vi "DAQmx Data Acquisition.vi"(7 "measure call context in":refnum<class "Measure Call Context.lvclass">, 8 "error in":errorcluster, 11 "DAQmx Cfg":T1={"Run Mode"=0, "Sample Rate (Hz)"=51200.0, "Block Size"=5120, "Channel Table"=[], "Trigger Type"=0, "Trigger Channel"="", "Level"=0.0, "Pretrigger"=20, "Hysteresis"=0.0, "Slope"=enum."Rising"} {"Run Mode" items=["Run Once", "Continuously"]; "Block Size" min=0; "Sample Rate (Hz)" min=0.0; "Trigger Type" items=["None", "Analog Reference"]; "Channel Table"."input terminal configuration" items=["default"=-1, "RSE"=10083, "NRSE"=10078, "Differential"=10106, "Pseudodifferential"=12529]; "Channel Table"."Channel Type" items=["Voltage (V)"=0, "Charge (C)"=9, "-"=99, "SPL (Pa)"=3, "Force (lbf)"=6, "Force (N)"=1, "Acceleration (g) - IEPE"=2, "Acceleration (g) - Charge"=12, "Acceleration (g) - 4 wire DC Voltage"=22, "Velocity (in/s)"=7, "Velocity (mm/s)"=8, "Prox Probe (mil)"=4, "Prox Probe (mm)"=5]}) -> (0 "error out":errorcluster, 3 "waveforms channel":T4, 6 "stop channel":T3)   [LabVIEW 2024, in "DSA_CFG_ACQ.lvlib"]
doc: "Action engine that operates on DAQmx analog input task. The DAQmx task is created, configured, and managed in order to support data acquisition.\n\nNote: Triggering outputs discontinuous blocks of data (one new block per detected trigger). \n\nData is appended to the Waveform Data Buffer. \"New Data\" message is enqueued in the Marshalling Loop queue with current info as the message data."
uses:
  DSA_CFG_ACQ.lvlib
  <extravilib>/ChannelInstances/Messenger-a[.](wfm(dbl))/))Channel.ctl
  <vilib>/Plug-In SDKs/Measurements/Measure Call Context/Measure Call Context.lvclass
  <extravilib>/ChannelInstances/Tag-bool/))Channel.ctl
  Dynamic Signal Acquisition (Interactive) UI/SFPDAQ Configuration.ctl
  Dynamic Signal Acquisition (Interactive) UI/SFPDAQmx Channel Info.ctl
  controls/SFPDAQ States.ctl
  <vilib>/addons/Sound and Vibration/svt_DAQmx/subVIs/Device Info.ctl
  controls/SFPLogging Info.ctl
  8bc0de78-1497-4bf9-bc5e-99b3f246cc49.vi/ff40df25-0e41-4205-825d-56c19dc320b6.vi
  <vilib>/addons/_NISVFA/_Shared subVIs/Common/svc_Temperature in deg C to String.vi
  <vilib>/addons/_NISVFA/_Shared subVIs/Common/svc_Calibration Timestamp and Temperature to String.vi
  <vilib>/addons/_NISVFA/_Shared subVIs/Groups/SV Get Software Trigger Parameters.vi
  <extravilib>/ChannelInstances/Tag-bool/Read.vi
  <extravilib>/ChannelInstances/Tag-bool/Write.vi
  <vilib>/addons/_NISVFA/_Shared subVIs/Common/sv_Get NI Property Name String.vi
  <vilib>/addons/_NISVFA/_Shared subVIs/Common/sv_Get SV Property Name String.vi
  <extravilib>/ChannelInstances/Tag-bool/Read With Abort.vi
  <vilib>/Utility/Debug Log/Display.vi
  <vilib>/Plug-In SDKs/Measurements/Measure Call Context/Update Results.vi
  <vilib>/DAQmx/miscellaneous.llb/DAQmx Fill In Error Info.vi
  <vilib>/addons/_NISVFA/_Shared subVIs/Groups/SV Software Triggering (Analog Edge).vi
  <extravilib>/ChannelInstances/Messenger-a[.](wfm(dbl))/Endpoint.vi
  <extravilib>/ChannelInstances/Tag-bool/EndpointRead.vi
  <extravilib>/ChannelInstances/Tag-bool/Endpoint.vi
  Dynamic Signal Acquisition (Interactive) UI/Dynamic Signal Acquisition (Interactive) UI.lvlib
  Dynamic Signal Acquisition (Interactive).lvlib
  <vilib>/addons/Sound and Vibration/svt_DAQmx/subVIs/SV_DAQmx.lvlib
  <extravilib>/ChannelInstances/Messenger-a[.](wfm(dbl)).lvlib
  <extravilib>/ChannelInstances/Tag-bool.lvlib
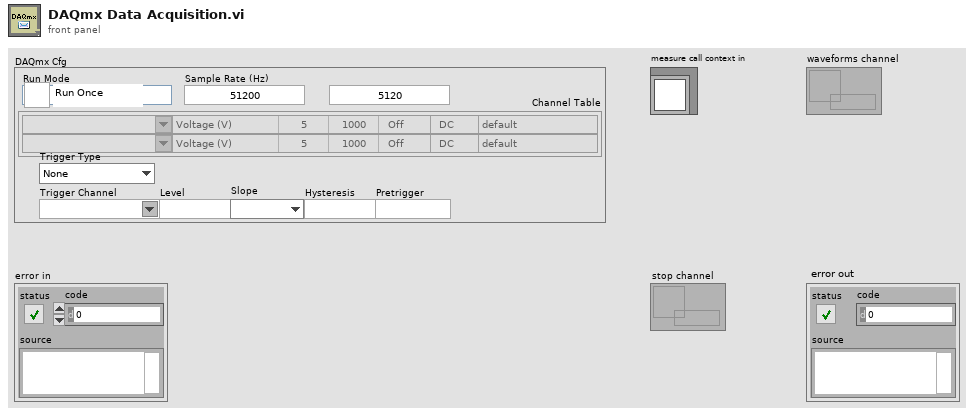
[diagram p1: front panel]
types:
  T1 = typedef "Dynamic Signal Acquisition (Interactive) UI.lvlib/SFPDAQ Configuration.ctl" = cluster{"Run Mode":u16, "Sample Rate (Hz)":dbl, "Block Size":i32, "Channel Table":T2[], "Trigger Type":u16, "Trigger Channel":string, "Level":dbl, "Pretrigger":i32, "Hysteresis":dbl, "Slope":enum16{"Falling", "Rising"}}
  T2 = typedef "Dynamic Signal Acquisition (Interactive) UI.lvlib/SFPDAQmx Channel Info.ctl" = cluster{"DAQmx Channel":tag, "Channel Type":u16, "Max":dbl, "Sensitivity":dbl, "Coupling":enum16{"AC", "DC"}, "input terminal configuration":i32, "excitation":enum16{"Off", "Min", "Max"}}
  T3 = typedef "Tag-bool.lvlib/))Channel.ctl" = refnum<queue>
  T4 = typedef "Messenger-a[.](wfm(dbl)).lvlib/))Channel.ctl" = refnum<queue>
  T5 = typedef "Dynamic Signal Acquisition (Interactive).lvlib/SFPDAQ States.ctl" = enum16{"Stopped", "Running"}
  T6 = typedef "SV_DAQmx.lvlib/Device Info.ctl" = cluster{"DAQmx Version":cluster{"Major":u32, "Minor":u32, "Update":u32}, "Time Stamp":timestamp, "Device Info":cluster{"Device":tag, "Product Type":string, "Serial Number":u32, "Current Temperature":dbl, "External Calibration Timestamp":timestamp, "External Calibration Temperature":dbl, "Self Calibration Timestamp":timestamp, "Self Calibration Temperature":dbl}[]}
  T7 = typedef "Dynamic Signal Acquisition (Interactive).lvlib/SFPLogging Info.ctl" = cluster{"enabled":bool, "file path":path, "timestamp":timestamp, "elapsed time":dbl}
  T8 = cluster{"AI Task":refnum<k21>, "State":T5, "Force Trigger":bool, "device info":T6, "logging info":T7, "DAQmx Cfg":T1, "log duration":dbl, "log directory":path, "log folder name":string, "dummy name":string, "name format":string, "read timeout":dbl, "read samples":i32, "update interval":dbl}
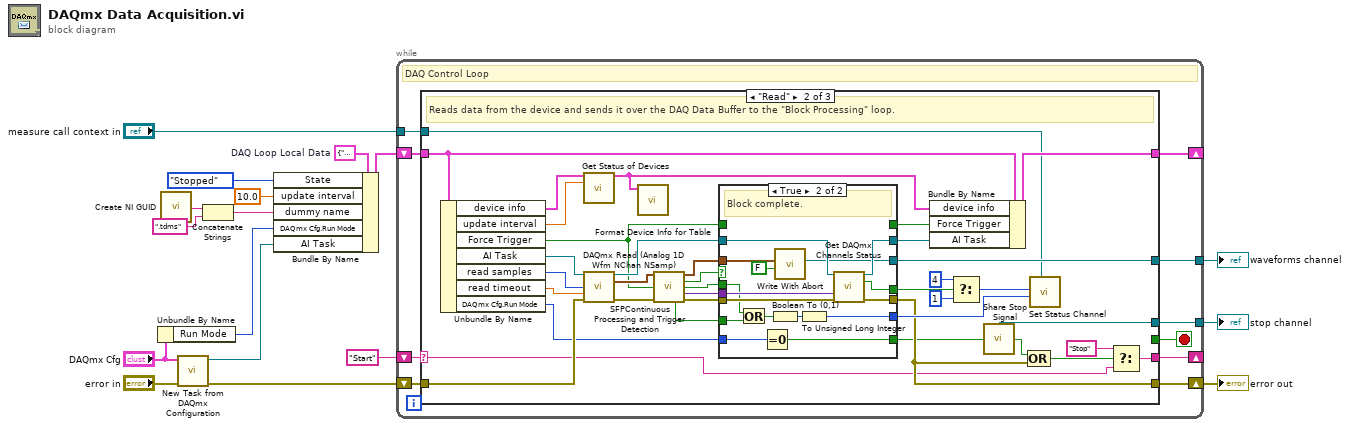
[diagram p0: block diagram]
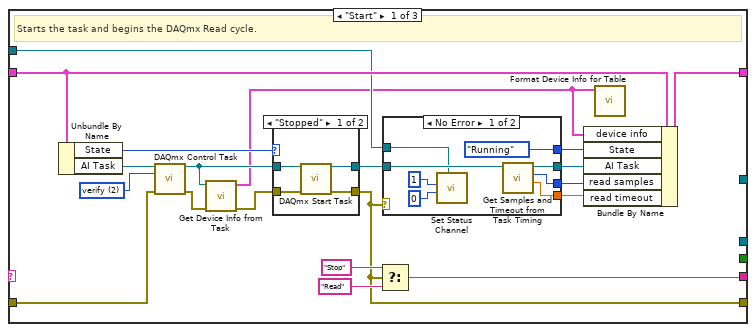
[diagram p2: hidden frame]
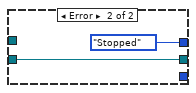
[diagram p4: hidden frame]
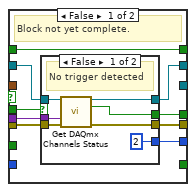
[diagram p5: hidden frame]
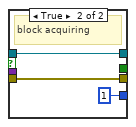
[diagram p6: hidden frame]
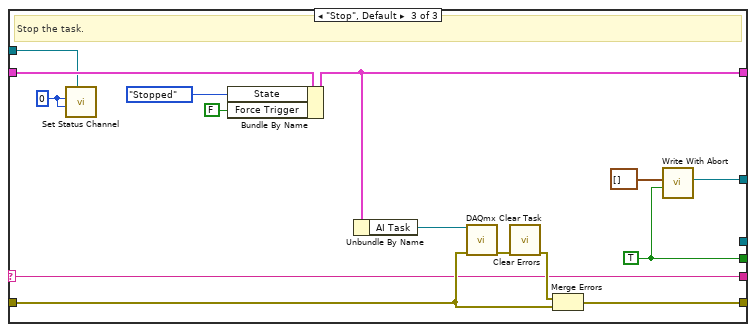
[diagram p7: hidden frame]
diagram:
  w17 = T8 {"AI Task"="", "State"=enum."Stopped", "Force Trigger"=FALSE, "device info"={"DAQmx Version"={"Major"=0, "Minor"=0, "Update"=0}, "Time Stamp"=timestamp(0 s since 1904-01-01), "Device Info"=[]}, "logging info"={"enabled"=FALSE, "file path"=path "", "timestamp"=timestamp(0 s since 1904-01-01), "elapsed time"=0.0}, "DAQmx Cfg"={"Run Mode"=1, "Sample Rate (Hz)"=51200.0, "Block Size"=5120, "Channel Table"=[], "Trigger Type"=0, "Trigger Channel"="", "Level"=1.0, "Pretrigger"=1, "Hysteresis"=0.0, "Slope"=enum."Rising"}, "log duration"=0.0, "log directory"=path "", "log folder name"="Recordings", "dummy name"="deleteme.tdms", "name format"="%Y%m%d_%H%M%S.tdms", "read timeout"=0.0, "read samples"=0, "update interval"=0.0}  # DAQ Loop Local Data
  n1 = Unbundle By Name("DAQmx Cfg") -> ("Run Mode"=w1:u16)
  n2 = call <vilib>:"Create NI GUID.vi"() -> ("NI GUID"=w13:string)
  n3 = call "New Task from DAQmx Configuration.vi"("error in"="error in", "DAQmx Cfg"="DAQmx Cfg") -> ("error out"=w5:errorcluster, "DAQmx task"=w3:refnum<k21>)  [unwired: 8 in]
  n4 = Concatenate Strings(w13, ".tdms" ("dummy file name")) -> (w8:string)
  n5 = Bundle By Name(cluster=w17, "State"=SFPDAQ_States."Stopped", "update interval"=10.0, "dummy name"=w8, "DAQmx Cfg.Run Mode"=w1, "AI Task"=w3) -> (w16:T8)
  n6 = while "DATA ACQUISITION (DAQ) and CONTINUOUS PROCESSING: Event-Gated Action Engine to Acquire Analog Input Data and Apply Continuous Processing. Produces Block Data" {
    shift-right: [w24] -> w11
    shift-left: w5 -> [w20]
    shift-right: [w26] -> _
    shift-left: w16 -> [w27]
    tunnel: [w25] -> w14
    tunnel: "measure call context in" -> [w23]
    tunnel: "stop channel" -> [w22]
    shift-right: [w18] -> _
    shift-left: "Start" ("Message") -> [w19]
    stop <- w21 stop-if-true
    # "DAQ Control Loop"
    n7 = case shown="\"Read\"" w19 {
      selector: w19 -> [_ w65 w136]
      tunnel: [_ _ w143] -> w21
      tunnel: w20 -> [w40 w98 w146]
      tunnel: [w29 w69 w145] -> w24
      tunnel: w27 -> [w39 w100 w150]
      tunnel: [w43 w99 w137] -> w26
      tunnel: [_ w80 w142] -> w25
      tunnel: w23 -> [w35 w75 w141]
      tunnel: w22 -> [_ w74 _]
      tunnel: [w30 w66 w136] -> w18
      frame "Start" {
        w44 = 2 items=["verify"=2, "reserve"=4, "commit"=3, "unreserve"=5, "abort"=6] ("action")
        # "Starts the task and begins the DAQmx Read cycle."
        n8 = Unbundle By Name(w39) -> ("State"=w36:T5, "AI Task"=w34:refnum<k21>)
        n9 = call <vilib>:"DAQmx Control Task.vi"("task/channels in"=w34, "action"=w44, "error in"=w40) -> ("task out"=w33:refnum<k21>, "error out"=w45:errorcluster)  [unwired: 11 in]
        n10 = call <vilib>:"Get Device Info from Task.vi"("error in"=w45, "task"=w33) -> ("error out"=w46:errorcluster, "device info out"=w28:T6)  [unwired: 8 in]
        n11 = case shown="\"Stopped\"" w36 {
          tunnel: w46 -> [w51 w53]
          tunnel: [w50 w53] -> w29
          tunnel: w33 -> [w49 w52]
          tunnel: [w48 w52] -> w47
          frame "Stopped" {
            n12 = call <vilib>:"DAQmx Start Task.vi"("task/channels in"=w49, "error in"=w51) -> ("task out"=w48:refnum<k21>, "error out"=w50:errorcluster)  [unwired: 12 in]
          }
          frame "Running" {
          }
        }
        n13 = Select(t="Stop", s=w29, f="Read") -> (s? t:f=w30:string)
        n14 = case shown="No Error" w29 {
          tunnel: w47 -> [w58 w62]
          tunnel: [SFPDAQ_States."Running" ("State") SFPDAQ_States."Stopped" ("State")] -> w42
          tunnel: [w59 w62] -> w41
          tunnel: [w57 _] -> w38
          tunnel: [w56 _] -> w37
          tunnel: w35 -> [w54 _]
          frame No Error {
            n15 = call "Set Status Channel.vi"("measure call context in"=w54, "trigger"=u16 0, "channels"=u16 1 ("task")) -> ()  [unwired: 9 in]
            n16 = call "Get Samples and Timeout from Task Timing.vi"("task in"=w58) -> ("timeout"=w57:dbl, "samples"=w56:i32, "task out"=w59:refnum<k21>)  [unwired: 7 in, 1 out]
          }
          frame Error {
          }
        }
        n17 = Bundle By Name(cluster=w39, "device info"=w28, "State"=w42, "AI Task"=w41, "read samples"=w37, "read timeout"=w38) -> (w43:T8)
        n18 = call <vilib>:"Format Device Info for Table.vi"("device info"=w28) -> ()  [unwired: 10 in, 1 out]
      }
      frame "Read" {
        # "Reads data from the device and sends it over the DAQ Data Buffer to the \"Block Processing\" loop."
        n19 = Unbundle By Name(w100) -> ("device info"=w90:T6, "update interval"=w76:dbl, "Force Trigger"=w68:bool, "AI Task"=w91:refnum<k21>, "read samples"=w78:i32, "read timeout"=w77:dbl, "DAQmx Cfg.Run Mode"=w72:u16)
        n20 = call <vilib>:"Get Status of Devices.vi"("device info"=w90, "update interval"=w76) -> ("device info"=w64:T6)  [unwired: 12 in, 1 out]
        n21 = call <vilib>:"DAQmx Read (Analog 1D Wfm NChan NSamp).vi"("task/channels in"=w91, "number of samples per channel"=w78, "timeout"=w77, "error in"=w98) -> ("task out"=w88:refnum<k21>, "data"=w97:waveform(dbl)[], "error out"=w86:errorcluster)  [unwired: 9 in]
        n22 = call <vilib>:"Format Device Info for Table.vi"("device info"=w64) -> ()  [unwired: 10 in, 1 out]
        n23 = call "SFPContinuous Processing and Trigger Detection.vi"("Input Signals"=w97, "force trigger (F)"=w68, "error in (no error)"=w86) -> ("signals"=w96:waveform(dbl)[], "signal available"=w95:bool, "new trigger detected"=w93:bool, "status info out"=w92:variant, "trigger enabled"=w85:bool, "error out"=w94:errorcluster)  [unwired: 7 in]
        n24 = case "triggered data ready?" shown="True" w95 {
          tunnel: w93 -> [w109 w129]
          tunnel: w96 -> [_ w135]
          tunnel: w94 -> [w104 w133]
          tunnel: [w103 w130] -> w69
          tunnel: w92 -> [w108 w134]
          tunnel: w72 -> [_ w121]
          tunnel: [w106 w131] -> w89
          tunnel: w88 -> [w107 w132]
          tunnel: [w105 _] -> w87
          tunnel: w68 -> [w105 _]
          tunnel: w85 -> [_ w128]
          tunnel: [w101 w122] -> w84
          tunnel: [w102 w127] -> w82
          tunnel: [_ w126] -> w80
          tunnel: [_ w120] -> w67
          frame False {
            # "Block not yet complete."
            n25 = case shown="False" w109 {
              tunnel: w108 -> [w116 _]
              tunnel: w107 -> [w115 w119]
              tunnel: [w114 w119] -> w106
              tunnel: w104 -> [w113 w118]
              tunnel: [w110 w118] -> w103
              tunnel: [w112 _] -> w102
              tunnel: [u32 2 ("task") u32 1 ("Task")] -> w101
              frame False {
                # "No trigger detected"
                n26 = call "Get DAQmx Channels Status.vi"("DAQmx task"=w115, "status info in"=w116, "error in"=w113) -> ("DAQmx task"=w114:refnum<k21>, "channel errors"=w112:bool, "error out"=w110:errorcluster)  [unwired: 9 in, 1 out]
              }
              frame True {
                # "block acquiring"
              }
            }
          }
          frame True {
            # "Block complete."
            n27 = Or(x=w129, y=w128) -> (x .or. y?=w123:bool)
            n28 = Equal To 0?(x=w121) -> (x = 0?=w120:bool)
            n29 = Boolean To (0,1)(Boolean=w123) -> (0, 1=w124:i16)
            n30 = call <extravilib>:"Write With Abort.vi"("abort (F)"=FALSE, "element"=w135) -> ("channel"=w126:T4)  [unwired: 6 in, 3 out]
            n31 = To Unsigned Long Integer(number=w124) -> (unsigned 32bit integer=w122:u32)
            n32 = call "Get DAQmx Channels Status.vi"("DAQmx task"=w132, "status info in"=w134, "error in"=w133) -> ("DAQmx task"=w131:refnum<k21>, "channel errors"=w127:bool, "error out"=w130:errorcluster)  [unwired: 9 in, 1 out]
          }
        }
        n33 = Bundle By Name(cluster=w100, "device info"=w64, "Force Trigger"=w87, "AI Task"=w89) -> (w99:T8)
        n34 = Select(t=u32 4, s=w82, f=u32 1 ("Task")) -> (s? t:f=w81:u32)
        n35 = call <vilib>:"Share Stop Signal.vi"("set stop (F)"=w67, "channel"=w74) -> ("stop"=w71:bool)
        n36 = Compound Arithmetic op=OR(w71, w69) -> (w70:bool)
        n37 = call "Set Status Channel.vi"("measure call context in"=w75, "trigger"=w84, "channels"=w81) -> ()  [unwired: 9 in]
        n38 = Select(t="Stop", s=w70, f=w65) -> (s? t:f=w66:string)
      }
      frame "Stop", Default {
        w140 = u16 0 ("channels")
        w143 = TRUE
        # "Stop the task."
        n39 = call "Set Status Channel.vi"("measure call context in"=w141, "trigger"=w140, "channels"=w140) -> ()  [unwired: 9 in]
        n40 = Bundle By Name(cluster=w150, "State"=SFPDAQ_States."Stopped", "Force Trigger"=FALSE) -> (w137:T8)
        n41 = Unbundle By Name(w137) -> ("AI Task"=w149:refnum<k21>)
        n42 = call <vilib>:"DAQmx Clear Task.vi"("task in"=w149, "error in"=w146) -> ("error out"=w139:errorcluster)  [unwired: 13 in]
        n43 = call <vilib>:"Clear Errors.vi"("error in (no error)"=w139) -> ("error out"=w138:errorcluster)  [unwired: 5 in, 1 out]
        n44 = Merge Errors(w138, w146) -> (w145:errorcluster)
        n45 = call <extravilib>:"Write With Abort.vi"("abort (F)"=w143, "element"=waveform(dbl)[] []) -> ("channel"=w142:T4)  [unwired: 6 in, 3 out]
      }
    }
  }
  "error out" <- w11
  "waveforms channel" <- w14
